vi "Feeder.vi"(10 "Power":dbl) -> ()   [LabVIEW 2016]
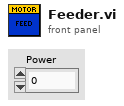
[diagram p1: front panel]
types:
  T1 = typedef "WPI_MotorControlDeviceRef.ctl" = cluster{"DeviceStatus":errorcluster, "Type":T2, "PWM":cluster{"PWM Channel":T3, "DeadBand":T4}, "CAN":cluster{"Device Number":u8, "SetOutput VI Ref":variant, "GetOutput VI Ref":variant, "Enable VI Ref":variant, "Disable VI Ref":variant, "Data":variant}, "Invert":bool}
  T2 = typedef "WPI_MotorControlType.ctl" = enum16{"PWM", "CAN"}
  T3 = typedef "FPGA_DIOPWMChannel.ctl" = enum8{"PWM 0", "PWM 1", "PWM 2", "PWM 3", "PWM 4", "PWM 5", "PWM 6", "PWM 7", "PWM 8", "PWM 9", "PWM MXP 0", "PWM MXP 1", "PWM MXP 2", "PWM MXP 3", "PWM MXP 4", "PWM MXP 5", "PWM MXP 6", "PWM MXP 7", "PWM MXP 8", "PWM MXP 9", "Invalid"}
  T4 = typedef "WPI_PWMDeadband.ctl" = cluster{"Name":string, "maxPositivePwm":i32, "minPositivePwm":i32, "centerPwm":i32, "maxNegativePwm":i32, "minNegativePwm":i32, "angularRange":u16}
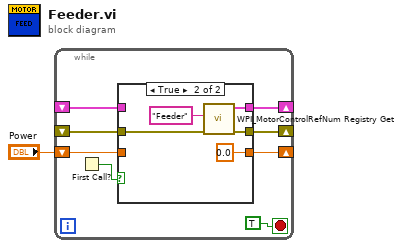
[diagram p0: block diagram]
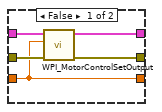
[diagram p2: hidden frame]
diagram:
  n1 = while {
    shift-right: [w5] -> _
    shift-left: _ -> [w7]
    shift-right: [w4] -> _
    shift-left: _ -> [w6]
    shift-right: [w2] -> _
    shift-left: "Power" -> [w3]
    stop <- TRUE stop-if-true
    n2 = First Call?() -> (First Call?: T/F=w8:bool)
    n3 = case shown="True" w8 {
      tunnel: w7 -> [w14 _]
      tunnel: w6 -> [w13 w17]
      tunnel: [w12 w18] -> w5
      tunnel: [w11 w16] -> w4
      tunnel: w3 -> [w10 _]
      tunnel: [w10 0.0 ("Power")] -> w2
      frame False {
        n4 = call <vilib>:"WPI_MotorControlSetOutput.vi"("error in (no error)"=w13, "Output"=w10, "MotorControlDevRef"=w14) -> ("error out"=w11:errorcluster, "MotorControlDevRef"=w12:T1)  [unwired: 6 in, 1 out]
      }
      frame True {
        n5 = call <vilib>:"WPI_MotorControlRefNum Registry Get.vi"("error in (no error)"=w17, "refnum name"="Feeder") -> ("error out"=w16:errorcluster, "MotorControlDevRef"=w18:T1)  [unwired: 8 in]
      }
    }
  }
